vi "Process.vi"(8 "error in":errorcluster, 11 "Plugin in":refnum<class "Digital Output Handler.lvclass">) -> (0 "error out":errorcluster, 3 "Plugin out":refnum<class "Digital Output Handler.lvclass">)   [LabVIEW 2023, in "Digital Output Handler.lvlib" / "Digital Output Handler.lvclass"]
uses:
  Digital Output Handler.lvclass
  C:/Program Files/National Instruments/LabVIEW 2023/vi.lib/FlexLogger/SDK/PluginSDK.lvlibp/PEFClasses/SDK/Plugin/Plugin.lvclass
  <vilib>/FlexLogger/SDK/PluginSDK.lvlibp/PEFClasses/SDK/Plugin/DataHelpers/Write 1D Bool (NChan 1 Sample).vi
  <vilib>/FlexLogger/SDK/PluginSDK.lvlibp/PEFClasses/SDK/Plugin/Plugin.lvclass
  C:/Program Files/National Instruments/LabVIEW 2023/vi.lib/FlexLogger/SDK/PluginSDK.lvlibp/PEFClasses/SDK/Processing Element/Processing Element.lvclass
  C:/Users/magranad/Documents/LabVIEW Projects/FlexLogger IO Plug-ins/Digital Output Handler/Digital Output Handler.lvclass
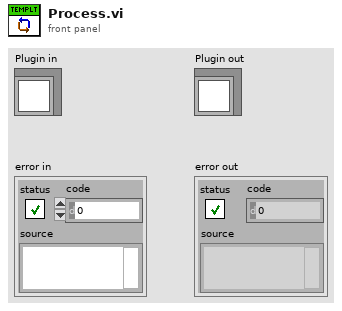
[diagram p1: front panel]
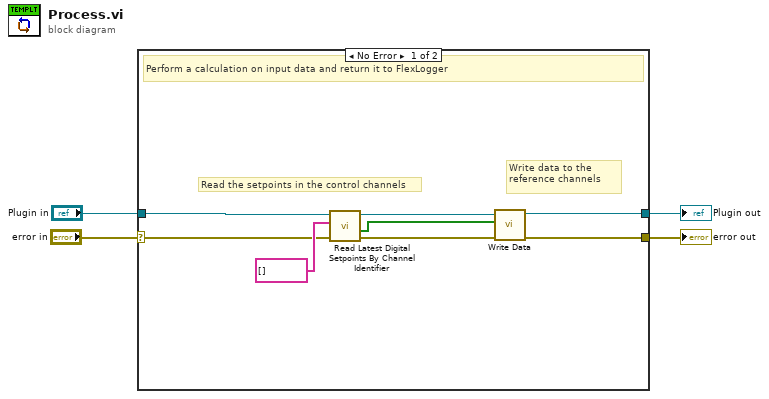
[diagram p0: block diagram]
diagram:
  n1 = case shown="No Error" "error in" {
    selector: "error in" -> [w6 w13]
    tunnel: [w11 w14] -> w1
    tunnel: "Plugin in" -> [w5 w14]
    tunnel: [w12 w13] -> w2
    frame No Error {
      # "Read the setpoints in the control channels"
      # "Write data to the reference channels"
      # "Perform a calculation on input data and return it to FlexLogger"
      n2 = call <vilib>:"Read Latest Digital Setpoints By Channel Identifier.vi"("error in (no error)"=w6, "Unique Channel Identifers (empty = all)"=string[] [], "Plugin in"=w5) -> ("error out"=w7:errorcluster, "Values"=w9:bool[], "Plugin out"=w8:refnum<class "Digital Output Handler.lvclass">)  [unwired: 5 in, 1 out]
      n3 = call-poly <vilib>:"Write Data.vi"("error in (no error)"=w7, "Data"=w9, "Plugin in"=w8) -> ("error out"=w12:errorcluster, "Plugin out"=w11:refnum<class "Digital Output Handler.lvclass">)  [unwired: 7 in]
    }
    frame Error {
    }
  }
  "error out" <- w2
  "Plugin out" <- w1
